vi "ConvertToAbsolute.vi"(11 "Yaw":dbl) -> (3 "Absolute Yaw":dbl)   [LabVIEW 2015, in "Nav6.lvlib"]
uses:
  Nav6.lvlib
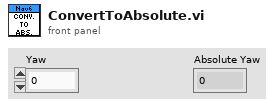
[diagram p1: front panel]
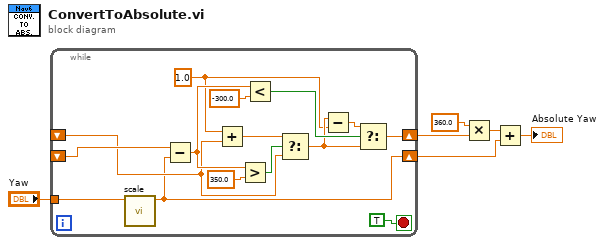
[diagram p0: block diagram]
diagram:
  n1 = while {
    shift-right: [w7] -> w1
    shift-left: _ -> [w16]
    tunnel: "Yaw" -> [w20]
    shift-right: [w15] -> w2
    shift-left: _ -> [w12]
    stop <- TRUE stop-if-true
    w9 = 1.0 ("x")
    n2 = call "scale.vi"("Yaw"=w20) -> ("Scaled Yaw"=w7:dbl)  [unwired: 10 in]
    n3 = Subtract(x=w16, y=w7) -> (x-y=w14:dbl)
    n4 = Add(x=w9, y=w12) -> (x+y=w10:dbl)
    n5 = Greater?(x=w14, y=350.0) -> (0:w17:bool)
    n6 = Less?(x=w14, y=-300.0) -> (x < y?=w13:bool)
    n7 = Select(t=w10, s=w17, f=w12) -> (s? t:f=w11:dbl)
    n8 = Subtract(x=w11, y=w9) -> (x-y=w8:dbl)
    n9 = Select(t=w8, s=w13, f=w11) -> (s? t:f=w15:dbl)
  }
  n10 = Multiply(x=360.0, y=w2) -> (x*y=w4:dbl)
  n11 = Add(x=w4, y=w1) -> (x+y=→"Absolute Yaw":dbl)
